vi "11.1.2.-Neurona Perceptrón.vi"() -> ()   [LabVIEW 2020]
panel:
  in  "T = Umbral de Activación":dbl[](array[numeric])
  out "a":bool
  in  "X2":dbl
  in  "X1":dbl
  out "XY Graph":cluster{dbl[], dbl[]}[](graph)
  # "Visión Artificial - Detección de Patrones - Neurona Perceptron\nDiego Cervantes Rodríguez\ndicer0.com"
  # "Patrones"
  # "Salida Deseada"
  # "Salida Obtenida"
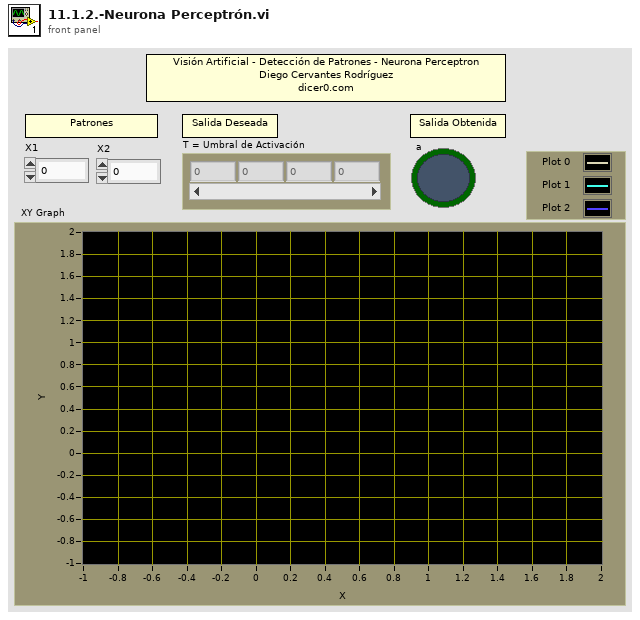
[diagram p1: front panel]
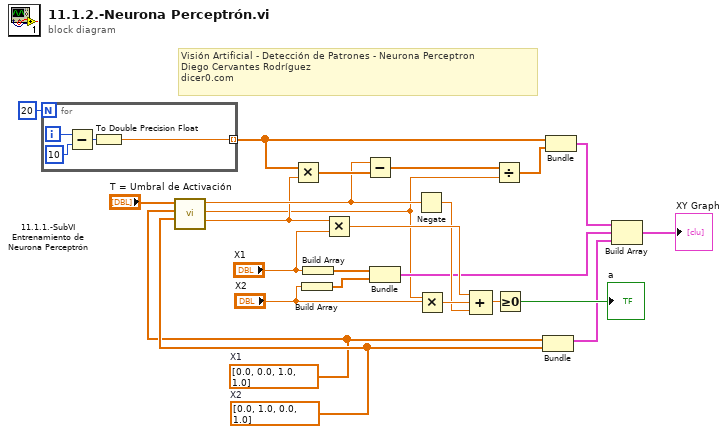
[diagram p0: block diagram]
diagram:
  w2 = dbl[] [0.0, 1.0, 0.0, 1.0]  # X2
  w1 = dbl[] [0.0, 0.0, 1.0, 1.0]  # X1
  # "Visión Artificial - Detección de Patrones - Neurona Perceptron\nDiego Cervantes Rodríguez\ndicer0.com"
  n1 = for {
    N: 20 -> [_]
    tunnel: [w25] -> w20 mode=indexing
    i -> [w28]
    n2 = Subtract(x=w28, y=10) -> (x-y=w26:i32)
    n3 = To Double Precision Float(number=w26) -> (double precision float=w25:dbl)
  }
  n4 = call "11.1.1.-SubVI Entrenamiento de Neurona Perceptrón.vi"("X2"=w2, "X1"=w1, "T = Umbral de Activación"="T = Umbral de Activación") -> ("W1"=w4:dbl, "W2"=w3:dbl, "B = Bias"=w5:dbl)  [unwired: 6 in]
  n5 = Multiply(x=w20, y=w4) -> (x*y=w23:dbl[])
  n6 = Build Array("X2") -> (w18:dbl[])
  n7 = Build Array "Build Array"("X1") -> (w19:dbl[])
  n8 = Multiply(x=w4, y="X1") -> (x*y=w13:dbl)
  n9 = Subtract(x=w5, y=w23) -> (x-y=w22:dbl[])
  n10 = Bundle "Bundle"(w19, w18) -> (w7:cluster{dbl[], dbl[]})  [unwired: 1 in]
  n11 = Negate(x=w5) -> (-x=w11:dbl)
  n12 = Multiply(x=w3, y="X2") -> (x*y=w12:dbl)
  n13 = Compound Arithmetic op=ADD(w13, w12, w11) -> (w10:dbl)
  n14 = Divide(x=w22, y=w3) -> (x/y=w21:dbl[])
  n15 = Greater Or Equal To 0?(x=w10) -> (x >= 0?=→"a":bool)
  n16 = Bundle("X1"=w1, "X2"=w2) -> (w8:cluster{"X1":dbl[], "X2":dbl[]})  [unwired: 1 in]
  n17 = Bundle "Bundle"(w20, w21) -> (w17:cluster{dbl[], dbl[]})  [unwired: 1 in]
  n18 = Build Array "Build Array"(w17, w7, w8) -> (→"XY Graph":cluster{"X1":dbl[], "X2":dbl[]}[])
